vi "write file with time.vi"(8 "error in":errorcluster, 10 "data":string) -> (0 "error out":errorcluster, 2 "data file path out":path)   [LabVIEW 2016]
doc: "This subvi writes a file with the given input and finds the correct direcotry to save it with custom *.txt file and the name of the file includes the date and time it was created.\n\nAlexis Lopez\nP350\nCSUSB Physics"
panel:
  in  "date format":enum16{"short", "long", "abbreviated"}(ring)
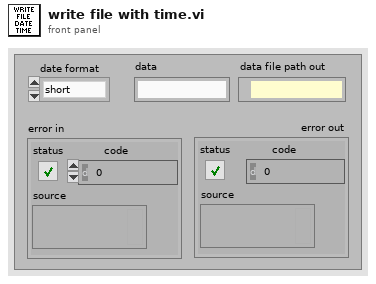
[diagram p1: front panel]
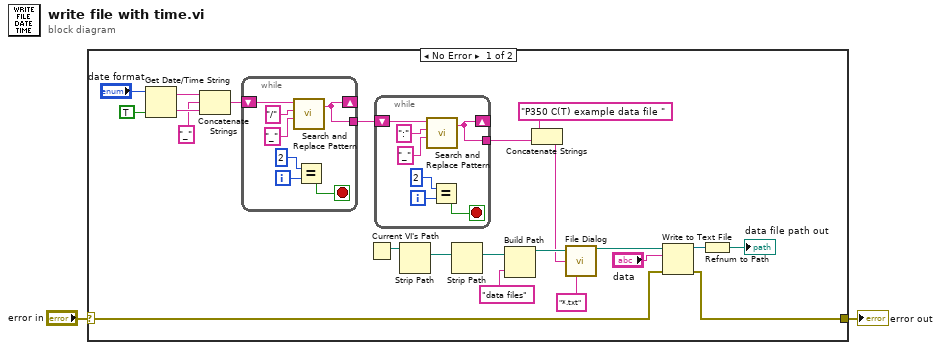
[diagram p0: block diagram]
diagram:
  n1 = case shown="No Error" "error in" {
    selector: "error in" -> [w6 w39]
    tunnel: [w5 w39] -> w1
    frame No Error {
      n2 = Get Date/Time String(date format (0)="date format", want seconds? (F)=TRUE) -> (date string=w22:string, time string=w19:string)  [unwired: 1 in]
      n3 = Concatenate Strings(w22, "_", w19) -> (w20:string)
      n4 = while {
        shift-right: [w37] -> _
        shift-left: w20 -> [w38]
        tunnel: [w37] -> w21
        i -> [w36]
        stop <- w34 stop-if-true
        n5 = call <vilib>:"Search and Replace Pattern.vi"("string"=w38, "regular expression (\"\")"="/", "replace string (\"\")"="_") -> ("result string"=w37:string)  [unwired: 2 in, 1 out]
        n6 = Equal?(x=2, y=w36) -> (x = y?=w34:bool)
      }
      n7 = Current VI's Path() -> (path=w17:path)
      n8 = while {
        shift-right: [w30] -> _
        shift-left: w21 -> [w31]
        tunnel: [w30] -> w14
        i -> [w27]
        stop <- w28 stop-if-true
        n9 = call <vilib>:"Search and Replace Pattern.vi"("string"=w31, "regular expression (\"\")"=":", "replace string (\"\")"="_") -> ("result string"=w30:string)  [unwired: 2 in, 1 out]
        n10 = Equal?(x=2, y=w27) -> (x = y?=w28:bool)
      }
      n11 = Strip Path(path=w17) -> (stripped path=w3:path)  [unwired: 1 out]
      n12 = Strip Path(path=w3) -> (stripped path=w4:path)  [unwired: 1 out]
      n13 = Build Path(base path=w4, name or relative path="data files") -> (appended path=w15:path)
      n14 = Concatenate Strings("P350 C(T) example data file ", w14) -> (w12:string)
      n15 = call "File Dialog"("start path"=w15, "default name"=w12, "pattern (all files)"="*.txt") -> ("selected path"=w10:path)  [unwired: 9 in, 3 out]
      n16 = Write to Text File(file (use dialog)=w10, text="data", error in=w6) -> (refnum out=w8:refnum<file>, error out=w5:errorcluster)  [unwired: 1 in, 1 out]
      n17 = Refnum to Path(1:w8) -> (0:→"data file path out":path)
    }
    frame Error {
    }
  }
  "error out" <- w1
